vi "Calibration_Save.vi"(0 "Img1":T3, 1 "Data":T1={"system"={"info"={"menuSelect"=0, "version"=0, "serial"="", "captureActive"=FALSE, "captureBegin"=FALSE, "emptyAndRefill"=FALSE}, "userInfo"={"operatorName"="", "date"=timestamp(2713993200 s since 1904-01-01)}, "camera"={"exposureTime"=0, "aperture"=enum."Item 0", "framerate"=0, "framerateMax"=500, "legacyAttributes"=FALSE}}, "connections"={"arduino"={"connection"="", "status"=FALSE, "openState"=FALSE, "emptyStart"=0}, "pump"={"connection"="MRJ", "status"=FALSE, "command"="", "dispenseSpeed"=100, "flushSize"=100}, "camera"={"cam1"={"connection"="", "status"=FALSE}, "cam2"={"connection"="", "status"=FALSE}}}, "queue"={"process"={"cam1"=refnum, "cam2"=refnum, "queueSize"=0}, "save"={"cam1"=refnum, "cam2"=refnum, "queueSize"=0}, "overloadThreshold"=0}, "imageProcess"={"cam1"={"preAllocation"={"image"="Station", "originalDisplay"="Station", "originalRgb"="Station", "binary"="Station", "save"="Station", "calibrationFull"=refnum, "calibrationDetect"=refnum}, "calibration"={"pathFull"=path "", "pathDetect"=path "", "ROI"={"Left"=0, "Top"=0, "Right"=0, "Bottom"=0, "Rotation"=0.0}}}, "cam2"={"preAllocation"={"image"=refnum, "originalDisplay"=refnum, "originalRgb"=refnum, "binary"=refnum, "save"=refnum, "calibrationFull"=refnum, "calibrationDetect"=refnum}, "calibration"={"pathFull"=path "C:/Users/au540322/Desktop/IHS_Project/images/Debris/Debris_0/Debris_0_2019_06_01-23-32-49-686.PNG", "pathDetect"=path "C:/Users/au540322/Desktop/IHS_Project/images/Debris/Debris_0/Debris_0_2019_06_01-23-32-49-686.PNG", "ROI"={"Left"=0, "Top"=0, "Right"=0, "Bottom"=0, "Rotation"=0.0}}}, "process"={"planeExtract"=refnum, "planeSubtract"=refnum, "cropMask"=refnum}, "detection"={"sampleTimeout"=500, "sizeThreshold"=500, "detectionRegionPct"=0.0}}, "sampleData"={"sampleId"="", "projectId"="", "voucherID"="", "speciesName"="", "collectionDate"=timestamp(2713993200 s since 1904-01-01), "sampleStation"="", "location"="", "lat"=0.0, "lon"=0.0, "determiner"="", "sex"="", "otherNotes"=""}, "Session In"=""} {"sampleData"."collectionDate" format="%<%Y-%m-%d>T"; "imageProcess"."detection"."sizeThreshold" min=1; "imageProcess"."cam2"."calibration"."ROI"."Rotation" format="%.2f"; "imageProcess"."cam2"."calibration"."ROI"."Left" scale=0.0..1024.0; "imageProcess"."cam2"."calibration"."ROI"."Right" scale=0.0..1024.0; "imageProcess"."cam1"."calibration"."ROI"."Rotation" format="%.2f"; "imageProcess"."cam1"."calibration"."ROI"."Left" scale=0.0..1024.0; "imageProcess"."cam1"."calibration"."ROI"."Right" scale=0.0..1024.0; "queue"."overloadThreshold" min=1; "queue"."save"."queueSize" min=1; "queue"."process"."queueSize" min=1; "connections"."pump"."flushSize" min=1; "connections"."pump"."dispenseSpeed" min=1; "system"."camera"."framerateMax" min=1; "system"."userInfo"."date" format="%<%Y-%m-%dT%H:%M:%S+%z>T"; "system"."info"."version" items=["Standard", "XL"]; "system"."info"."menuSelect" items=["Session Data", "Extended Setup", "Buffer", "Camera", "Dispenser", "Stats", "Connections"]}, 5 "Img2":T3, 9 "Dtct":bool, 11 "Crop?":bool) -> (4 "Cal1":path, 6 "Cal2":path, 8 "Data out":T1={"system"={"info"={"menuSelect"=0, "version"=0, "serial"="", "captureActive"=FALSE, "captureBegin"=FALSE, "emptyAndRefill"=FALSE}, "userInfo"={"operatorName"="", "date"=timestamp(2713993200 s since 1904-01-01)}, "camera"={"exposureTime"=0, "aperture"=enum."Item 0", "framerate"=0, "framerateMax"=500, "legacyAttributes"=FALSE}}, "connections"={"arduino"={"connection"="", "status"=FALSE, "openState"=FALSE, "emptyStart"=0}, "pump"={"connection"="MRJ", "status"=FALSE, "command"="", "dispenseSpeed"=100, "flushSize"=100}, "camera"={"cam1"={"connection"="", "status"=FALSE}, "cam2"={"connection"="", "status"=FALSE}}}, "queue"={"process"={"cam1"=refnum, "cam2"=refnum, "queueSize"=0}, "save"={"cam1"=refnum, "cam2"=refnum, "queueSize"=0}, "overloadThreshold"=0}, "imageProcess"={"cam1"={"preAllocation"={"image"="Station", "originalDisplay"="Station", "originalRgb"="Station", "binary"="Station", "save"="Station", "calibrationFull"=refnum, "calibrationDetect"=refnum}, "calibration"={"pathFull"=path "", "pathDetect"=path "", "ROI"={"Left"=0, "Top"=0, "Right"=0, "Bottom"=0, "Rotation"=0.0}}}, "cam2"={"preAllocation"={"image"=refnum, "originalDisplay"=refnum, "originalRgb"=refnum, "binary"=refnum, "save"=refnum, "calibrationFull"=refnum, "calibrationDetect"=refnum}, "calibration"={"pathFull"=path "C:/Users/au540322/Desktop/IHS_Project/images/Debris/Debris_0/Debris_0_2019_06_01-23-32-49-686.PNG", "pathDetect"=path "C:/Users/au540322/Desktop/IHS_Project/images/Debris/Debris_0/Debris_0_2019_06_01-23-32-49-686.PNG", "ROI"={"Left"=0, "Top"=0, "Right"=0, "Bottom"=0, "Rotation"=0.0}}}, "process"={"planeExtract"=refnum, "planeSubtract"=refnum, "cropMask"=refnum}, "detection"={"sampleTimeout"=500, "sizeThreshold"=500, "detectionRegionPct"=0.0}}, "sampleData"={"sampleId"="", "projectId"="", "voucherID"="", "speciesName"="", "collectionDate"=timestamp(2713993200 s since 1904-01-01), "sampleStation"="", "location"="", "lat"=0.0, "lon"=0.0, "determiner"="", "sex"="", "otherNotes"=""}, "Session In"=""} {"sampleData"."collectionDate" format="%<%Y-%m-%d>T"; "imageProcess"."detection"."sizeThreshold" min=1; "imageProcess"."cam2"."calibration"."ROI"."Rotation" format="%.2f"; "imageProcess"."cam2"."calibration"."ROI"."Left" scale=0.0..1024.0; "imageProcess"."cam2"."calibration"."ROI"."Right" scale=0.0..1024.0; "imageProcess"."cam1"."calibration"."ROI"."Rotation" format="%.2f"; "imageProcess"."cam1"."calibration"."ROI"."Left" scale=0.0..1024.0; "imageProcess"."cam1"."calibration"."ROI"."Right" scale=0.0..1024.0; "queue"."overloadThreshold" min=1; "queue"."save"."queueSize" min=1; "queue"."process"."queueSize" min=1; "connections"."pump"."flushSize" min=1; "connections"."pump"."dispenseSpeed" min=1; "system"."camera"."framerateMax" min=1; "system"."userInfo"."date" format="%<%Y-%m-%dT%H:%M:%S+%z>T"; "system"."info"."version" items=["Standard", "XL"]; "system"."info"."menuSelect" items=["Session Data", "Extended Setup", "Buffer", "Camera", "Dispenser", "Stats", "Connections"]}, 10 "Img1 out":T3, 15 "Img2 out":T3)   [LabVIEW 2022 SP3]
uses:
  controls/Data.ctl
  <vilib>/userdefined/High Color/IMAQdx.ctl
  <vilib>/vision/Image Controls.llb/IMAQ Image.ctl
panel:
  out "error out 2":errorcluster
  out "error out":errorcluster
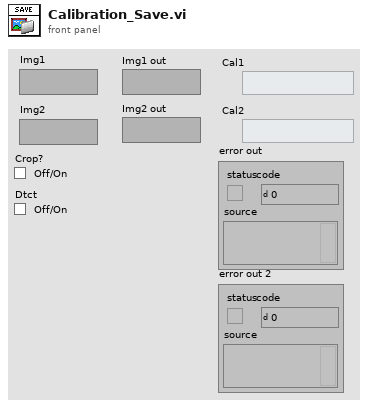
[diagram p1: front panel]
types:
  T1 = typedef "Data.ctl" = cluster{"system":cluster{"info":cluster{"menuSelect":u16, "version":u16, "serial":string, "captureActive":bool, "captureBegin":bool, "emptyAndRefill":bool}, "userInfo":cluster{"operatorName":string, "date":timestamp}, "camera":cluster{"exposureTime":i32, "aperture":enum32{"Item 0", "Item 1", "Item 2", "Item 3"}, "framerate":i32, "framerateMax":i32, "legacyAttributes":bool}}, "connections":cluster{"arduino":cluster{"connection":refnum<visa-resource-name>, "status":bool, "openState":bool, "emptyStart":u32}, "pump":cluster{"connection":refnum<visa-resource-name>, "status":bool, "command":string, "dispenseSpeed":i32, "flushSize":i32}, "camera":cluster{"cam1":cluster{"connection":T2, "status":bool}, "cam2":cluster{"connection":T2, "status":bool}}}, "queue":cluster{"process":cluster{"cam1":refnum<queue>, "cam2":refnum<queue>, "queueSize":i32}, "save":cluster{"cam1":refnum<queue>, "cam2":refnum<queue>, "queueSize":i32}, "overloadThreshold":i32}, "imageProcess":cluster{"cam1":cluster{"preAllocation":cluster{"image":T3, "originalDisplay":T3, "originalRgb":T3, "binary":T3, "save":T3, "calibrationFull":T3, "calibrationDetect":T3}, "calibration":cluster{"pathFull":path, "pathDetect":path, "ROI":T4}}, "cam2":cluster{"preAllocation":cluster{"image":T3, "originalDisplay":T3, "originalRgb":T3, "binary":T3, "save":T3, "calibrationFull":T3, "calibrationDetect":T3}, "calibration":cluster{"pathFull":path, "pathDetect":path, "ROI":T4}}, "process":cluster{"planeExtract":T3, "planeSubtract":T3, "cropMask":T3}, "detection":cluster{"sampleTimeout":i32, "sizeThreshold":i32, "detectionRegionPct":dbl}}, "sampleData":cluster{"sampleId":string, "projectId":string, "voucherID":string, "speciesName":string, "collectionDate":timestamp, "sampleStation":string, "location":string, "lat":dbl, "lon":dbl, "determiner":string, "sex":string, "otherNotes":string}, "Session In":T2}
  T2 = typedef "IMAQdx.ctl" = refnum<k21>
  T3 = typedef "IMAQ Image.ctl" = refnum<image>
  T4 = typedef "IMAQ Rectangle" = cluster{"Left":i32, "Top":i32, "Right":i32, "Bottom":i32, "Rotation":dbl}
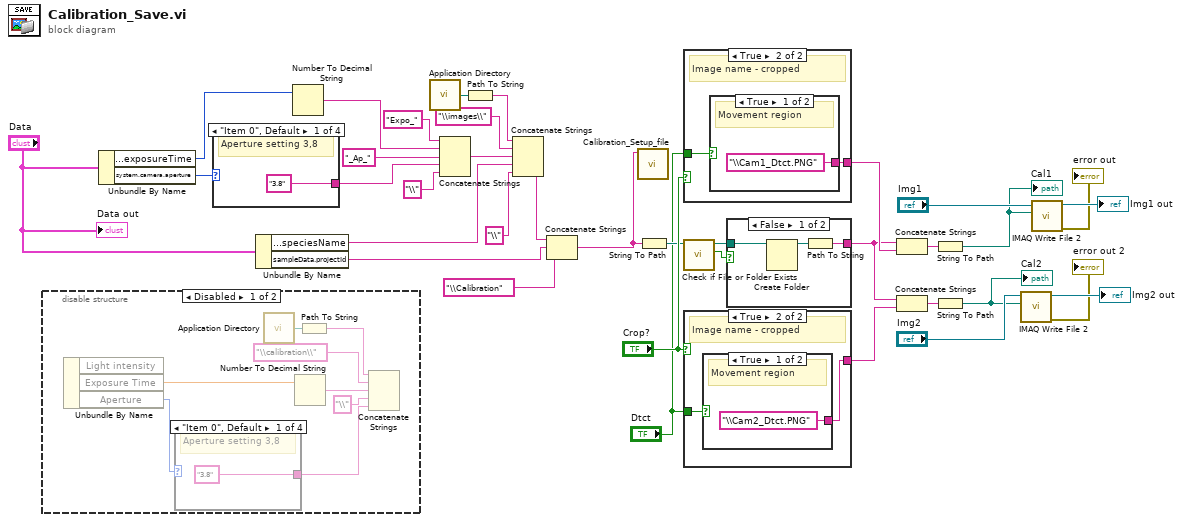
[diagram p0: block diagram]
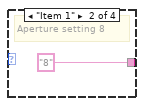
[diagram p2: hidden frame]
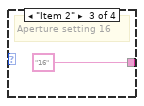
[diagram p3: hidden frame]
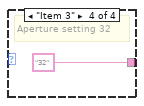
[diagram p4: hidden frame]
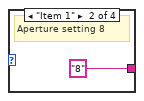
[diagram p6: hidden frame]
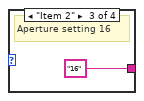
[diagram p7: hidden frame]
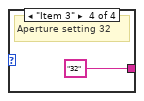
[diagram p8: hidden frame]
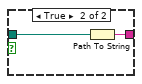
[diagram p9: hidden frame]
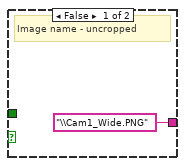
[diagram p10: hidden frame]
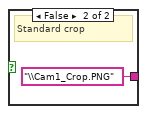
[diagram p11: hidden frame]
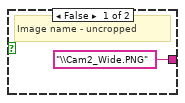
[diagram p12: hidden frame]
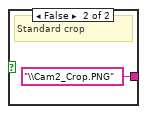
[diagram p13: hidden frame]
diagram:
  n1 = disable-structure shown="Disabled" {
    frame Disabled {
      n2 = Unbundle By Name() -> ("Exposure Time"=w43:dbl, "Aperture"=w37:enum32{"Item 0", "Item 1", "Item 2", "Item 3"})  [unwired: 1 in, 1 out]
      n3 = case shown="\"Item 0\", Default" w37 {
        tunnel: ["3.8" "8" "16" "32"] -> w38
        frame "Item 0", Default {
          # "Aperture setting 3,8"
        }
        frame "Item 1" {
          # "Aperture setting 8"
        }
        frame "Item 2" {
          # "Aperture setting 16"
        }
        frame "Item 3" {
          # "Aperture setting 32"
        }
      }
      n4 = call <vilib>:"Application Directory.vi"() -> ("Application Directory"=w40:path)
      n5 = Number To Decimal String(number=w43) -> (decimal integer string=w42:string)  [unwired: 1 in]
      n6 = Path To String(path=w40) -> (string=w39:string)
      n7 = Concatenate Strings(w39, "\\calibration\\" ("string"), w42, "\\" ("string"), w38) -> ()  [unwired: 1 out]
    }
    frame Enabled {
    }
  }
  n8 = Unbundle By Name("Data") -> ("system.camera.exposureTime"=w21:i32, "system.camera.aperture"=w18:enum32{"Item 0", "Item 1", "Item 2", "Item 3"})
  n9 = case shown="\"Item 0\", Default" w18 {
    tunnel: ["3.8" "8" "16" "32"] -> w16
    frame "Item 0", Default {
      # "Aperture setting 3,8"
    }
    frame "Item 1" {
      # "Aperture setting 8"
    }
    frame "Item 2" {
      # "Aperture setting 16"
    }
    frame "Item 3" {
      # "Aperture setting 32"
    }
  }
  n10 = Unbundle By Name("Data") -> ("sampleData.speciesName"=w25:string, "sampleData.projectId"=w23:string)
  n11 = Number To Decimal String(number=w21) -> (decimal integer string=w17:string)  [unwired: 1 in]
  n12 = call <vilib>:"Application Directory.vi"() -> ("Application Directory"=w26:path)
  n13 = Concatenate Strings("Expo_" ("string"), w17, "_Ap_" ("string"), w16, "\\" ("string")) -> (w14:string)
  n14 = Path To String(path=w26) -> (string=w27:string)
  n15 = Concatenate Strings(w27, "\\images\\" ("string"), w14, w25, "\\" ("string")) -> (w24:string)
  n16 = Concatenate Strings(w24, w23, "\\Calibration" ("string")) -> (w13:string)
  n17 = call "Calibration_Setup_file.vi"("Path"=w13) -> ()  [unwired: 11 in]
  n18 = String To Path(string=w13) -> (path=w31:path)
  n19 = case shown="True" "Crop?" {
    tunnel: ["\\Cam1_Wide.PNG" ("string") w55] -> w35
    tunnel: "Dtct" -> [_ w54]
    frame False {
      # "Image name - uncropped"
    }
    frame True {
      # "Image name - cropped"
      n20 = case shown="True" w54 {
        tunnel: ["\\Cam1_Dtct.PNG" ("string") "\\Cam1_Crop.PNG" ("string")] -> w55
        frame True {
          # "Movement region"
        }
        frame False {
          # "Standard crop"
        }
      }
    }
  }
  n21 = call <vilib>:"Check if File or Folder Exists.vi"("path"=w31) -> ("file or folder exists?"=w33:bool, "dup path"=w32:path)  [unwired: 8 in, 1 out]
  n22 = case shown="True" "Crop?" {
    tunnel: ["\\Cam2_Wide.PNG" ("string") w60] -> w36
    tunnel: "Dtct" -> [_ w59]
    frame False {
      # "Image name - uncropped"
    }
    frame True {
      # "Image name - cropped"
      n23 = case shown="True" w59 {
        tunnel: ["\\Cam2_Dtct.PNG" ("string") "\\Cam2_Crop.PNG" ("string")] -> w60
        frame True {
          # "Movement region"
        }
        frame False {
          # "Standard crop"
        }
      }
    }
  }
  n24 = case shown="False" w33 {
    tunnel: w32 -> [w65 w67]
    tunnel: [w63 w66] -> w30
    frame False {
      n25 = Create Folder(path (use dialog)=w65) -> (created path=w64:path)  [unwired: 2 in, 2 out]
      n26 = Path To String(path=w64) -> (string=w63:string)
    }
    frame True {
      n27 = Path To String(path=w67) -> (string=w66:string)
    }
  }
  n28 = Concatenate Strings(w30, w35) -> (w9:string)
  n29 = Concatenate Strings(w30, w36) -> (w10:string)
  n30 = String To Path(string=w9) -> (path=w6:path)
  "Cal1" <- w6
  n31 = String To Path(string=w10) -> (path=w5:path)
  "Cal2" <- w5
  n32 = call-poly "IMAQ Write File 2"("File Path"=w5, "Image"="Img2") -> ("error out"=→"error out 2":errorcluster, "Image Out (duplicate)"=→"Img2 out":T3)  [unwired: 8 in]
  n33 = call-poly "IMAQ Write File 2"("File Path"=w6, "Image"="Img1") -> ("error out"=→"error out":errorcluster, "Image Out (duplicate)"=→"Img1 out":T3)  [unwired: 8 in]
  "Data out" <- "Data"
